vi "AP2_doubling_spline_generation.vi"() -> ()   [LabVIEW 2023]
panel:
  in  "Main Control Tab":enum32{"Controls", "Monitoring"}(tab)
  in  "stop":bool
  in  "Step Size / nm":dbl
  in  "Lower Bound / nm":dbl
  in  "Upper bound / nm":dbl
  in  "Start Optimisation":bool
  in  "Cancel Optimisation":bool
  in  "BBO Motor Step Size":i32
  in  "BBO Start Position":i32
  in  "Initial Step Direction":u16
  in  "Averaging Time / s":u32
  out "RT Laser Power / J":dbl
  out "XY Graph":cluster{dbl[], dbl[]}(graph)
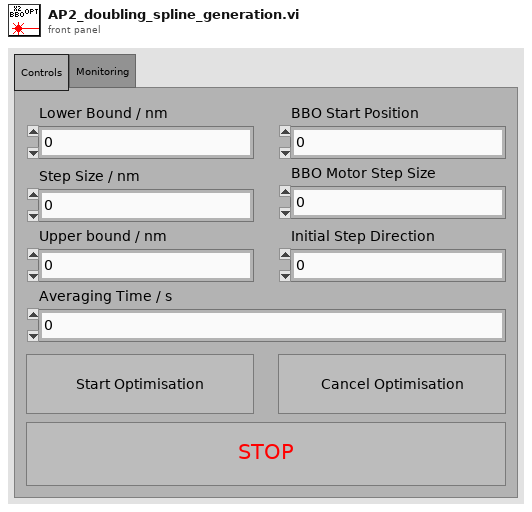
[diagram p1: front panel]
types:
  T1 = cluster{"queue out":refnum<queue>, "error out":errorcluster}
  T2 = cluster{"OphirLMMeasurementLib.ICoLMMeasurement2":refnum<k7>, "Error":errorcluster, "hDevice":i32}
  T3 = cluster{"BBO Start Position":i32, "Step Size":i32, "Initial Step Direction":u16, "Averaging Time / s ":u32}
  T4 = cluster{"Upper bound":dbl, "Step Size":dbl, "Lower Bound":dbl}
  T5 = cluster{"Power Reading ":dbl, "T imestamp":dbl, "Status":i32}
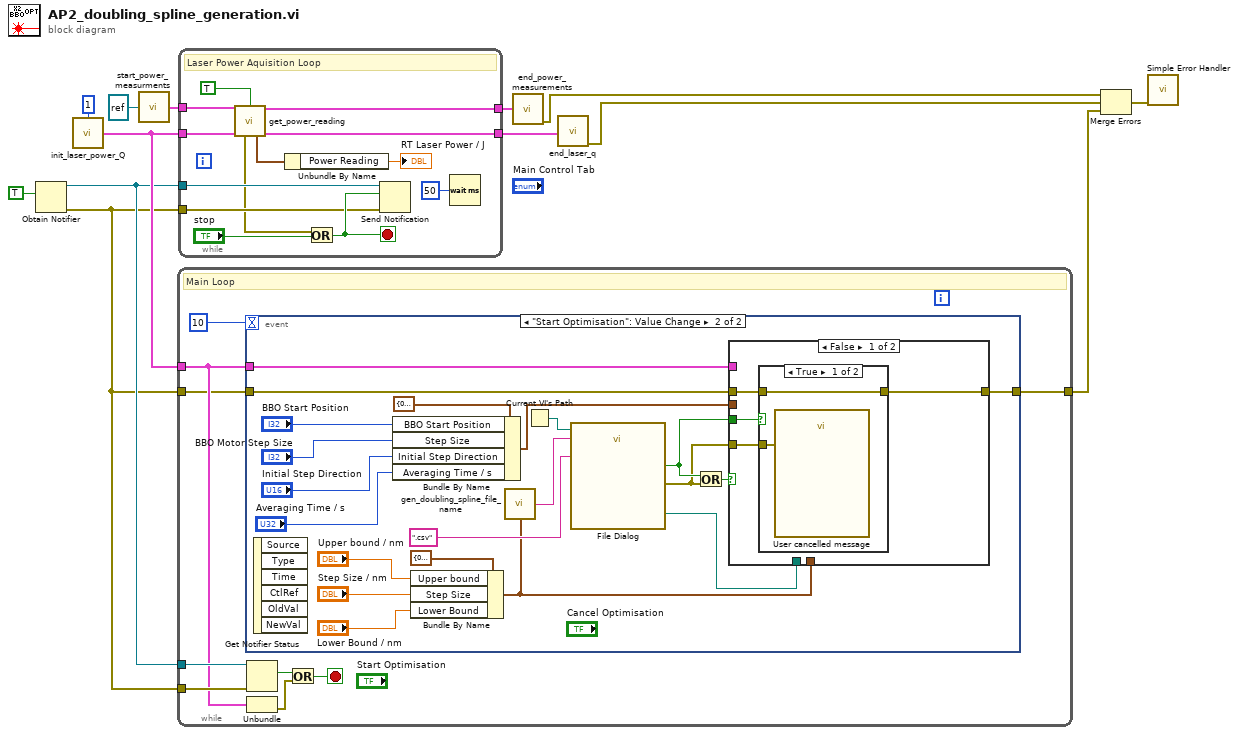
[diagram p0: block diagram]
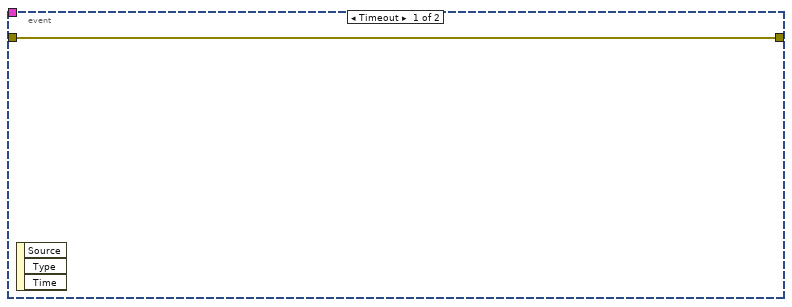
[diagram p2: hidden frame]
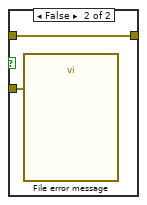
[diagram p3: hidden frame]
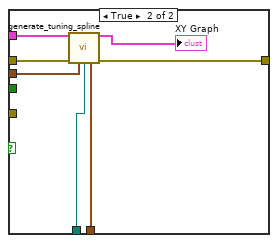
[diagram p4: hidden frame]
diagram:
  n1 = Obtain Notifier(notification data type=TRUE) -> (notifier out=w7:refnum<notifier>, error out=w5:errorcluster)  [unwired: 3 in, 1 out]
  n2 = call "init_laser_power_Q.vi"("max queue size (-1, unlimited)"=1) -> ("Laser Power Q"=w9:T1)  [unwired: 14 in]
  n3 = call "start_power_measurments.vi"("OphirLMMeasurementLib.ICoLMMeasurement2"=refnum<k7> refnum) -> ("Power Meter Connection Data Out"=w13:T2)  [unwired: 14 in]
  n4 = while {
    tunnel: w9 -> [w16]
    tunnel: w7 -> [w21]
    tunnel: w5 -> [w20]
    tunnel: w5 -> [w15]
    tunnel: [w14] -> w2
    stop <- w19 stop-if-true
    # "Main Loop"
    n5 = event shown="[1] \"Start Optimisation\": Value Change" {
      selector: _ -> [_ _]
      dyn-events: _ -> [_ _]
      timeout: 10 -> [_ _]
      tunnel: w16 -> [_ w40]
      tunnel: w15 -> [w23 w39]
      tunnel: [w23 w38] -> w14
      event Timeout {
        n6 = event-data() -> ()  [unwired: 1 in, 3 out]
      }
      event "Start Optimisation": Value Change {
        n7 = event-data() -> ()  [unwired: 1 in, 6 out]
        n8 = Bundle By Name(cluster=T3 {"BBO Start Position"=0, "Step Size"=0, "Initial Step Direction"=0, "Averaging Time / s "=0} ("Controls Cluster"), "BBO Start Position"="BBO Start Position", "Step Size"="BBO Motor Step Size", "Initial Step Direction"="Initial Step Direction", "Averaging Time / s"="Averaging Time / s") -> (w32:T3)
        n9 = Bundle By Name(cluster=T4 {"Upper bound"=0.0, "Step Size"=0.0, "Lower Bound"=0.0}, "Upper bound"="Upper bound / nm", "Step Size"="Step Size / nm", "Lower Bound"="Lower Bound / nm") -> (w24:T4)
        n10 = call "gen_doubling_spline_file_name.vi"("output cluster"=w24) -> ("concatenated string"=w25:string)  [unwired: 14 in]
        n11 = Current VI's Path() -> (path=w27:path)
        n12 = call "File Dialog"("start path"=w27, "default name"=w25, "pattern (all files)"=".csv" ("pattern label")) -> ("selected path"=w30:path, "cancelled"=w29:bool, "error out"=w28:errorcluster)  [unwired: 9 in, 1 out]
        n13 = Or(x=w29, y=w28) -> (x .or. y?=w31:bool)
        n14 = case shown="False" w31 {
          tunnel: w40 -> [_ w59]
          tunnel: w24 -> [_ w55]
          tunnel: w39 -> [w48 w58]
          tunnel: [w47 w57] -> w38
          tunnel: w32 -> [_ w56]
          tunnel: w30 -> [_ w54]
          tunnel: w29 -> [w46 _]
          tunnel: w28 -> [w45 _]
          frame False {
            n15 = case shown="True" w46 {
              tunnel: w48 -> [w49 w51]
              tunnel: [w49 w51] -> w47
              tunnel: w45 -> [w50 w52]
              frame True {
                n16 = call "User cancelled message"("error in (no error)"=w50) -> ()  [unwired: 9 in, 2 out]
              }
              frame False {
                n17 = call "File error message"("error in (no error)"=w52) -> ()  [unwired: 9 in, 2 out]
              }
            }
          }
          frame True {
            n18 = call "generate_tuning_spline.vi"("Laser Power Q"=w59, "error in"=w58, "Controls Cluster"=w56, "file path (dialog if empty)"=w54, "Bounds"=w55) -> ("Opt Data"=→"XY Graph":cluster{dbl[], dbl[]}, "error out"=w57:errorcluster)  [unwired: 9 in]
          }
        }
      }
    }
    n19 = Get Notifier Status(notifier=w21, error in (no error)=w20) -> (current notification=w18:bool)  [unwired: 4 out]
    n20 = Unbundle(w16) -> ("error out"=w17:errorcluster)  [unwired: 1 out]
    n21 = Or(x=w18, y=w17) -> (x .or. y?=w19:bool)
  }
  n22 = while {
    tunnel: w13 -> [w71]
    tunnel: w9 -> [w70]
    tunnel: [w69] -> w11
    tunnel: [w68] -> w10
    tunnel: w7 -> [w65]
    tunnel: w5 -> [w64]
    stop <- w66 stop-if-true
    # "Laser Power Aquisition Loop"
    n23 = call "get_power_reading.vi"("Power Meter Connection Data In"=w71, "Q Laser Data?"=TRUE, "Laser Power Q In"=w70) -> ("Power Meter Connection Data Out"=w69:T2, "error out"=w61:errorcluster, "Data Out"=w62:T5, "Laser Power Q Out"=w68:T1)  [unwired: 9 in]
    n24 = Unbundle By Name(w62) -> ("Power Reading"=→"RT Laser Power / J":dbl)
    n25 = Or(x=w61, y="stop") -> (x .or. y?=w66:bool)
    n26 = Send Notification(notification=w66, notifier=w65, error in (no error)=w64) -> ()  [unwired: 2 out]
    n27 = Wait (ms)(milliseconds to wait=u32 50) -> ()  [unwired: 1 out]
  }
  n28 = call "end_power_measurements.vi"("Power Meter Connection Data In"=w11) -> ("error out"=w4:errorcluster)  [unwired: 14 in]
  n29 = call "end_laser_q.vi"("Laser Power Q In"=w10) -> ("error out"=w3:errorcluster)  [unwired: 14 in]
  n30 = Merge Errors(w4, w3, w2) -> (w1:errorcluster)
  n31 = call <vilib>:"Simple Error Handler.vi"("error in (no error)"=w1) -> ()  [unwired: 4 in, 5 out]
